vi "FPGA_CounterWriteConfiguration.vi"(1 "Enable":bool, 4 "IndexActiveHigh":bool=TRUE, 5 "IndexSource":T1={"DevStatus"={"status"=FALSE, "code"=0, "source"=""}, "AnalogTriggerMode?"=FALSE, "DigitalMode"={"DIO Channel"=enum."Disabled"}, "AnalogTriggerMode"={"AnalogTriggerIndex"=enum."Trig 0", "OutputType"=enum."InWindow"}}, 6 "GTSDirThreshold":sgl, 7 "EdgeType":T5={"Master Mode"=enum."Edge Detection", "UpChannel"=enum."Disabled", "DownChannel"=enum."Disabled", "High/Up"=FALSE}, 8 "error in (no error)":errorcluster, 9 "DownSource":T1={"DevStatus"={"status"=FALSE, "code"=0, "source"=""}, "AnalogTriggerMode?"=FALSE, "DigitalMode"={"DIO Channel"=enum."Disabled"}, "AnalogTriggerMode"={"AnalogTriggerIndex"=enum."Trig 0", "OutputType"=enum."InWindow"}}, 10 "UpSource":T1={"DevStatus"={"status"=FALSE, "code"=0, "source"=""}, "AnalogTriggerMode?"=FALSE, "DigitalMode"={"DIO Channel"=enum."Disabled"}, "AnalogTriggerMode"={"AnalogTriggerIndex"=enum."Trig 0", "OutputType"=enum."InWindow"}}, 11 "Ctr Ref in":T6={"DevStatus"={"status"=FALSE, "code"=0, "source"=""}, "CntIndex"=enum."Ctr 1"}) -> (0 "error out":errorcluster, 3 "Ctr Ref out":T6={"DevStatus"={"status"=FALSE, "code"=0, "source"=""}, "CntIndex"=enum."Ctr 1"})   [LabVIEW 2017]
uses:
  <vilib>/Rock Robotics/SystemInterfaces/Counter/FPGA_CounterCtrDevRef.ctl
  <vilib>/Rock Robotics/SystemInterfaces/Counter/FPGA_CounterCtrSystemIndex.ctl
  <vilib>/Rock Robotics/SystemInterfaces/Counter/FPGA_CounterCtrEdgeDetectionType.ctl
  <vilib>/Rock Robotics/SystemInterfaces/CounterEncoderSourceConvertion/FPGA_CounterEncoderSourceConvertionLVSourceType.ctl
  <vilib>/Rock Robotics/SystemInterfaces/DIO/FPGA_DIODigitalSourceChannel.ctl
  <vilib>/Rock Robotics/SystemInterfaces/AnalogTrigger/FPGA_AnalogTriggerIndex.ctl
  <vilib>/Rock Robotics/SystemInterfaces/AnalogTrigger/FPGA_AnalogTriggerOutType.ctl
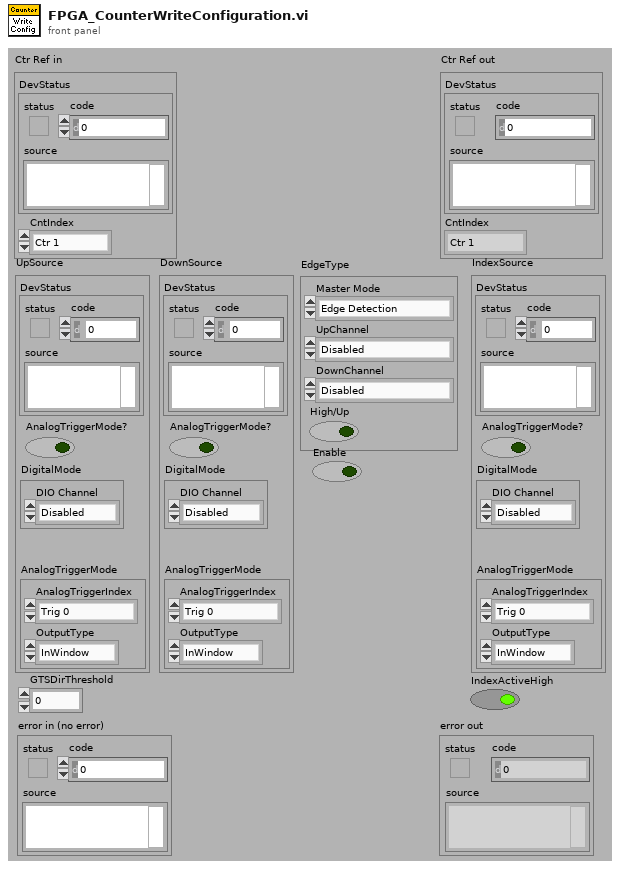
[diagram p1: front panel]
types:
  T1 = typedef "FPGA_CounterEncoderSourceConvertionLVSourceType.ctl" = cluster{"DevStatus":errorcluster, "AnalogTriggerMode?":bool, "DigitalMode":cluster{"DIO Channel":T2}, "AnalogTriggerMode":cluster{"AnalogTriggerIndex":T3, "OutputType":T4}}
  T2 = typedef "FPGA_DIODigitalSourceChannel.ctl" = enum8{"DIO 0", "DIO 1", "DIO 2", "DIO 3", "DIO 4", "DIO 5", "DIO 6", "DIO 7", "DIO 8", "DIO 9", "DIO MXP 0", "DIO MXP 1", "DIO MXP 2", "DIO MXP 3", "DIO MXP 4", "DIO MXP 5", "DIO MXP 6", "DIO MXP 7", "DIO MXP 8", "DIO MXP 9", "DIO MXP 10", "DIO MXP 11", "DIO MXP 12", "DIO MXP 13", "DIO MXP 14", "DIO MXP 15", "Disabled"}
  T3 = typedef "FPGA_AnalogTriggerIndex.ctl" = enum8{"Trig 0", "Trig 1", "Trig 2", "Trig 3", "Trig 4", "Trig 5", "Trig 6", "Trig 7", "Invalid"}
  T4 = typedef "FPGA_AnalogTriggerOutType.ctl" = enum16{"InWindow", "TriggerState", "Rising", "Falling"}
  T5 = typedef "FPGA_CounterCtrEdgeDetectionType.ctl" = cluster{"Master Mode":enum16{"Edge Detection", "Semi Period Mode", "Pulse Length Mode", "External Direction"}, "UpChannel":enum16{"Rising Edge", "Falling Edge", "Raising & Falling Edge", "Disabled"}, "DownChannel":enum16{"Rising Edge", "Falling Edge", "Raising & Falling Edge", "Disabled"}, "High/Up":bool}
  T6 = typedef "FPGA_CounterCtrDevRef.ctl" = cluster{"DevStatus":errorcluster, "CntIndex":T7}
  T7 = typedef "FPGA_CounterCtrSystemIndex.ctl" = enum8{"Ctr 0", "Ctr 1", "Ctr 2", "Ctr 3", "Ctr 4", "Ctr 5", "Ctr 6", "Ctr 7", "Invalid"}
  T8 = cluster{"Enable":bool, "UpSource":T1, "DownSource":T1, "IndexSource":T1, "IndexActiveHigh":bool, "EdgeType":T5, "GTSDirThreshold":sgl}
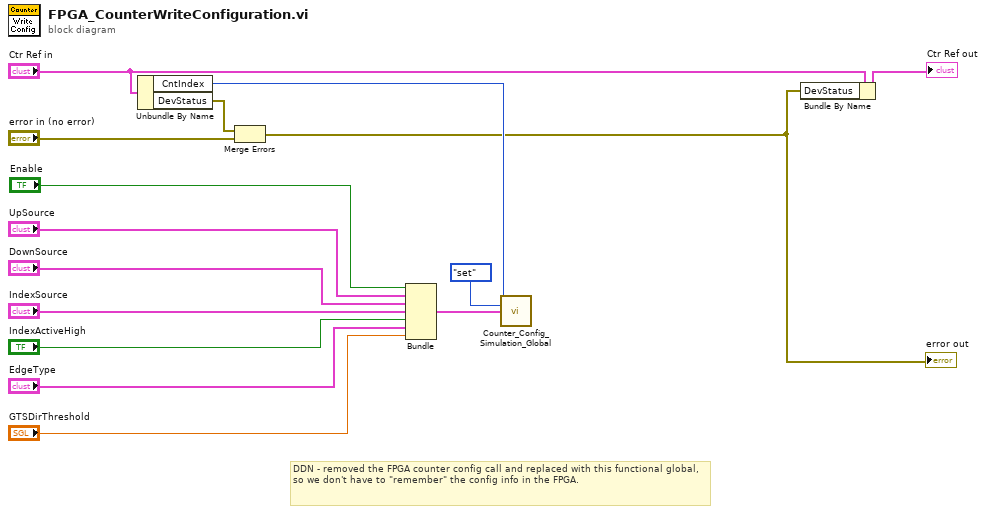
[diagram p0: block diagram]
diagram:
  # "DDN - removed the FPGA counter config call and replaced with this functional global, so we don't have to \"remember\" the config info in the FPGA."
  n1 = Unbundle By Name("Ctr Ref in") -> ("CntIndex"=w4:T7, "DevStatus"=w13:errorcluster)
  n2 = Merge Errors(w13, "error in (no error)") -> (w2:errorcluster)
  "error out" <- w2
  n3 = Bundle("Enable"="Enable", "UpSource"="UpSource", "DownSource"="DownSource", "IndexSource"="IndexSource", "IndexActiveHigh"="IndexActiveHigh", "EdgeType"="EdgeType", "GTSDirThreshold"="GTSDirThreshold") -> (w8:T8)  [unwired: 1 in]
  n4 = call <vilib>:"Counter_Config_Simulation_Global.vi"("CntIndex"=w4, "menu"=enum16{"set", "get", "delete"}."set", "ctr config set"=w8) -> ()  [unwired: 11 in, 2 out]
  n5 = Bundle By Name(cluster="Ctr Ref in", "DevStatus"=w2) -> (→"Ctr Ref out":T6)
